vi "stop.vi"(8 "error in (no error)":errorcluster, 11 "ExperimentControllerDL090130Interval in":refnum<class "ExperimentControllerDL090130Interval.lvclass">) -> (0 "error out":errorcluster, 3 "ExperimentControllerDL090130Interval out":refnum<class "ExperimentControllerDL090130Interval.lvclass">)   [LabVIEW 2010, in "ExperimentControllerDL090130Interval.lvclass"]
uses:
  ExperimentControllerDL090130Interval.lvclass
  schedule_entry_cluster.ctl
  internal_trigger_enum.ctl
  ExperimentControllerDL090130Interval.lvclass/ExperimentControllerDL090130Interval.ctl
  common/classes/ErrorController/ErrorController/class_data.vi
  common/classes/ErrorController/ErrorController/ErrorController.lvclass
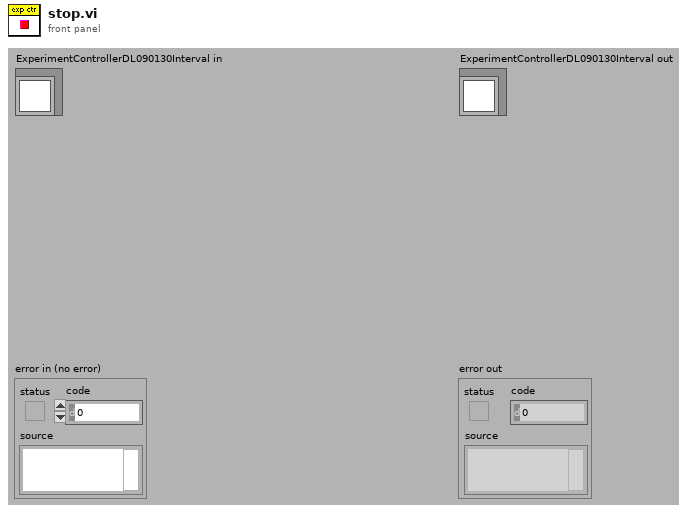
[diagram p1: front panel]
types:
  T1 = typedef "ExperimentControllerDL090130Interval.lvclass/schedule_entry_cluster.ctl" = cluster{"time":timestamp, "trigger":T2}
  T2 = typedef "ExperimentControllerDL090130Interval.lvclass/internal_trigger_enum.ctl" = enum16{"NULL", "initialise", "terminate", "start", "stop", "proceed", "prepare", "start sweep"}
  T3 = typedef "main_trigger_enum.ctl" = enum16{"NULL", "initialise", "terminate", "start", "stop", "change objective", "change experimentController", "change imagingMode", "save notebook", "started saving", "finished saving", "expCtr ready", "expCtr missing", "imgMd ready", "imgMd missing", "scanHd ready", "scanHd missing", "DAQ ready", "DAQ missing", "imgAsm ready", "imgAsm missing", "dataColl ready", "dataColl missing", "display ready", "display missing", "analysr ready", "analysr missing", "instrmnt ready", "instrmnt missing", "stimltr ready", "stimltr missing", "stage ready", "stage missing"}
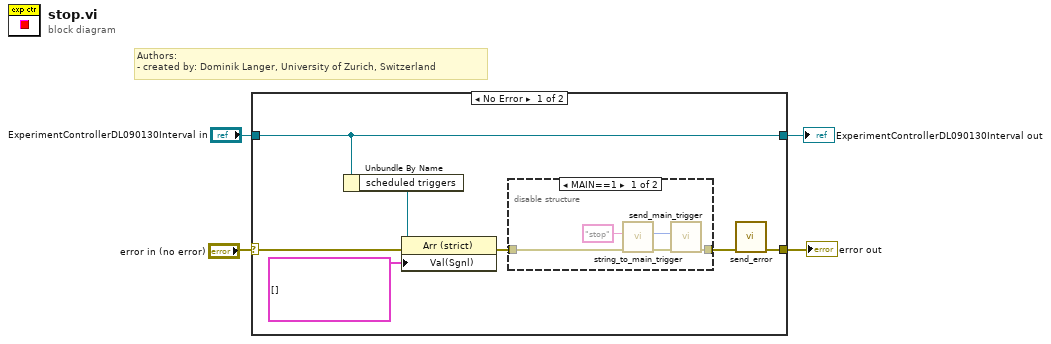
[diagram p0: block diagram]
diagram:
  # "Authors: \n- created by: Dominik Langer, University of Zurich, Switzerland"
  n1 = case shown="No Error" "error in (no error)" {
    selector: "error in (no error)" -> [w7 w19]
    tunnel: [w11 w19] -> w3
    tunnel: [w9 w18] -> w1
    tunnel: "ExperimentControllerDL090130Interval in" -> [w9 w18]
    frame No Error {
      n2 = Unbundle By Name(w9) -> ("scheduled triggers"=w8:refnum<vi>)
      n3 = property on="Property Node" class="Arr (strict)"(reference=w8, error in=w7, "Val(Sgnl)"=T1[] [] ("Value (Signaling)")) -> (error out=w6:errorcluster)  [unwired: 1 out]
      n4 = disable-structure shown="MAIN==1" {
        disable-tunnel: [w16 w17] -> w10
        disable-tunnel: w6 -> [w14 w17]
        frame condition #0 {
          n5 = call "string_to_main_trigger.vi"("error in (no error)"=w14, "trigger string"="stop") -> ("error out"=w13:errorcluster, "main trigger"=w12:T3)  [unwired: 8 in]
          n6 = call "send_main_trigger.vi"("error in (no error)"=w13, "trigger"=w12) -> ("error out"=w16:errorcluster)  [unwired: 9 in]
        }
        frame condition #1 (active) {
        }
      }
      n7 = call "send_error.vi"("error in (no error)"=w10) -> ("error out"=w11:errorcluster)  [unwired: 10 in]
    }
    frame Error {
    }
  }
  "error out" <- w3
  "ExperimentControllerDL090130Interval out" <- w1
